vi "Destroy Session.vi"(8 "error in (no error)":errorcluster, 11 "Session in":refnum<class "Session.lvclass">) -> (0 "error out":errorcluster, 3 "Session out":refnum<class "Session.lvclass">)   [LabVIEW 2020, in "HTTP Server.lvlib" / "Session.lvclass"]
uses:
  Session.lvclass
  Session.lvclass/Session.ctl
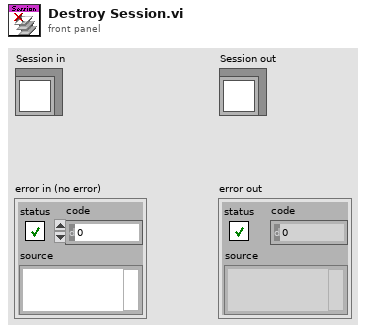
[diagram p1: front panel]
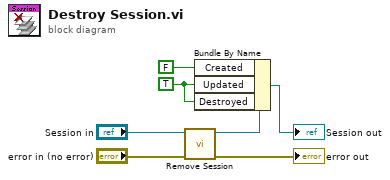
[diagram p0: block diagram]
diagram:
  w1 = TRUE ("Updated")
  n1 = call-dynamic "Remove Session.vi"("error in (no error)"="error in (no error)", "Session in"="Session in") -> ("error out"=→"error out":errorcluster, "Session out"=w5:refnum<class "Session.lvclass">)  [unwired: 8 in]
  n2 = Bundle By Name(cluster=w5, "Created"=FALSE, "Updated"=w1, "Destroyed"=w1) -> (→"Session out":refnum<class "Session.lvclass">)
